vi "Get VI Info.vi"(8 "error in":errorcluster, 11 "VI in":refnum<vi>) -> (0 "error out":errorcluster, 1 "VI Description":string, 2 "Plain Name":string, 3 "VI out":refnum<vi>, 4 "VI Path":path, 6 "VI Name":string)   [LabVIEW 2020, in "ConstantErrorsMaker.lvlib"]
uses:
  ConstantErrorsMaker.lvlib
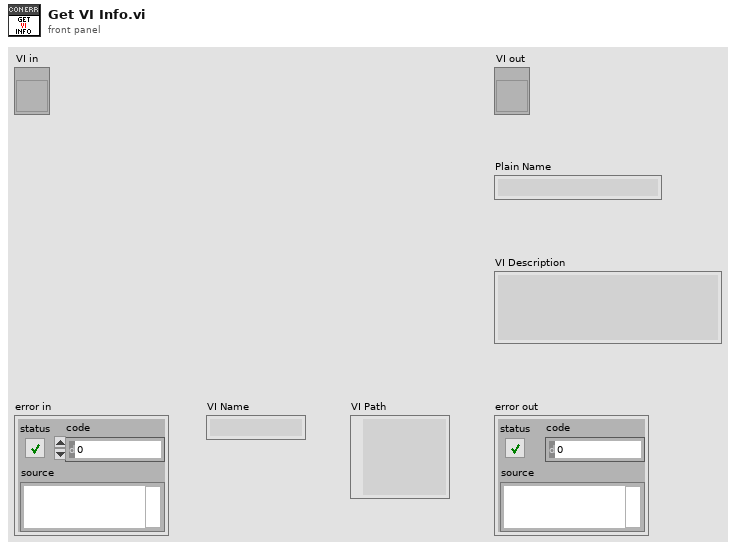
[diagram p1: front panel]
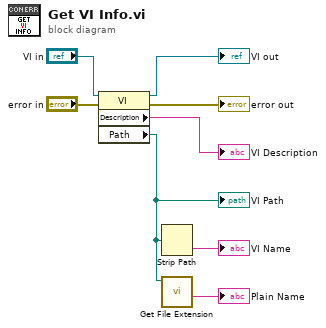
[diagram p0: block diagram]
diagram:
  n1 = property class="VI"(reference="VI in", error in="error in") -> (reference out=→"VI out":refnum<vi>, error out=→"error out":errorcluster, "Description"=→"VI Description":string, "Path"=w2:path)
  "VI Path" <- w2
  n2 = Strip Path(path=w2) -> (name=→"VI Name":string)  [unwired: 1 out]
  n3 = call <vilib>:"Get File Extension.vi"("file"=w2) -> ("filename without extension"=→"Plain Name":string)  [unwired: 6 in, 4 out]
